vi "Connect.vi"(8 "error in (no error)":errorcluster, 11 "Connection in":refnum<class "Connection.lvclass">) -> (0 "error out":errorcluster, 3 "Connection out":refnum<class "Connection.lvclass">)   [LabVIEW 2013, in "MQTT_Connection.lvlib" / "Connection.lvclass"]
uses:
  Connection.lvclass
  connection notifier.ctl
  Connection.lvclass/Connection.ctl
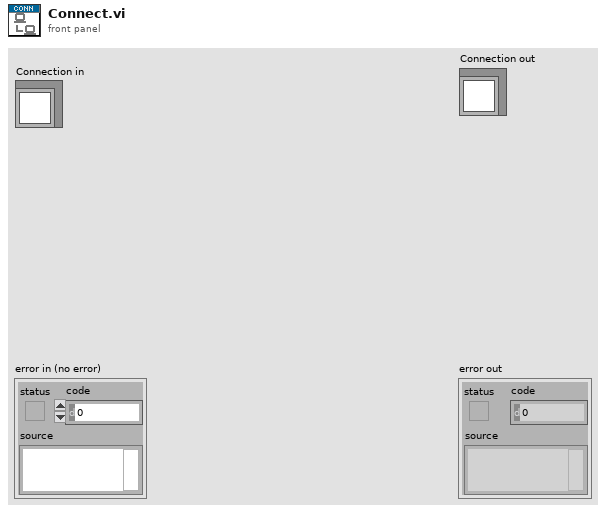
[diagram p1: front panel]
types:
  T1 = typedef "MQTT_Connection.lvlib/Connection.lvclass/connection notifier.ctl" = cluster{"Connection":refnum<class>, "error":errorcluster}
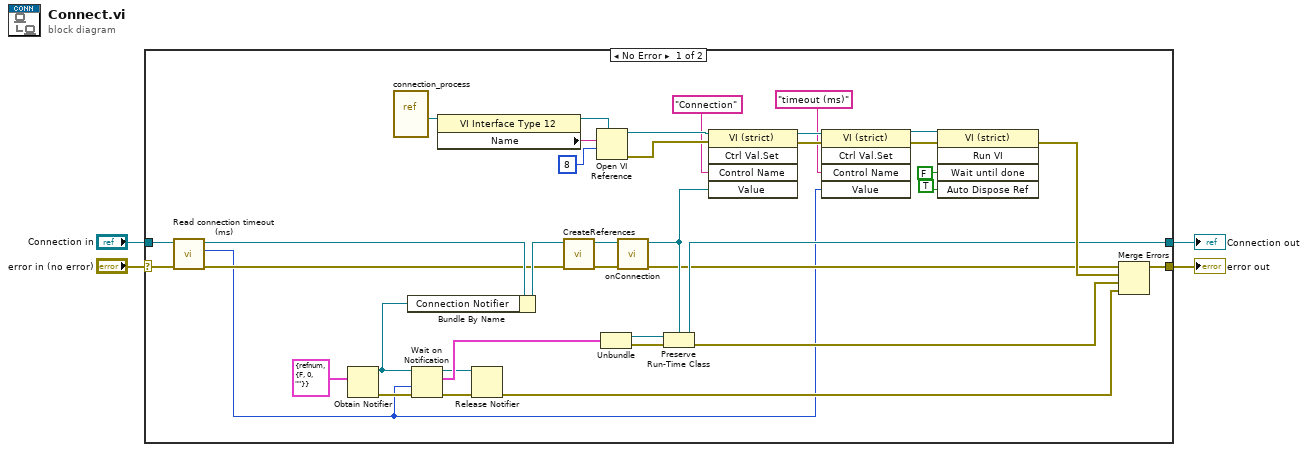
[diagram p0: block diagram]
diagram:
  n1 = case shown="No Error" "error in (no error)" {
    selector: "error in (no error)" -> [w7 w43]
    tunnel: [w39 w43] -> w3
    tunnel: [w14 w42] -> w2
    tunnel: "Connection in" -> [w9 w42]
    frame No Error {
      n2 = call "Read connection timeout (ms).vi"("error in (no error)"=w7, "Connection in"=w9) -> ("error out"=w6:errorcluster, "connection timeout (ms)"=w5:i32, "Connection out"=w8:refnum<class "Connection.lvclass">)  [unwired: 7 in]
      n3 = Obtain Notifier(notification data type=T1 {"Connection"=refnum, "error"={"status"=FALSE, "code"=0, "source"=""}} ("MQTT Server.lvlib:TCPConnection.lvclass:connection notifier")) -> (notifier out=w35:refnum<notifier>, error out=w41:errorcluster)  [unwired: 3 in, 1 out]
      n4 = vi-ref "connection_process.vi"() -> (w38:refnum<vi>)
      n5 = Bundle By Name(cluster=w8, "Connection Notifier"=w35) -> (w18:refnum<class "Connection.lvclass">)
      n6 = Wait on Notification(notifier=w35, timeout in ms (-1)=w5, error in (no error)=w41) -> (notifier out=w31:refnum<notifier>, notification=w40:T1, error out=w33:errorcluster)  [unwired: 1 in, 1 out]
      n7 = property class="VI Interface Type 12"(reference=w38) -> (reference out=w27:refnum<vi>, "Name"=w37:string)  [unwired: 1 in, 1 out]
      n8 = Release Notifier(notifier=w31, error in (no error)=w33) -> (error out=w32:errorcluster)  [unwired: 1 in, 2 out]
      n9 = call-dynamic "CreateReferences.vi"("error in (no error)"=w6, "Connection in"=w18) -> ("error out"=w11:errorcluster, "Connection out"=w13:refnum<class "Connection.lvclass">)  [unwired: 8 in]
      n10 = Open VI Reference(type specifier VI Refnum (for type only)=w27, vi path=w37, options=8) -> (vi reference=w30:refnum<vi>, error out=w29:errorcluster)  [unwired: 3 in]
      n11 = Unbundle(w40) -> ("Connection"=w17:refnum<class>, "error"=w16:errorcluster)
      n12 = call-dynamic "onConnection.vi"("error in (no error)"=w11, "Connection in"=w13) -> ("error out"=w10:errorcluster, "Connection out"=w12:refnum<class "Connection.lvclass">)  [unwired: 8 in]
      n13 = Preserve Run-Time Class(object in=w17, error in=w16, 2:w12) -> (object out=w14:refnum<class "Connection.lvclass">, error out=w15:errorcluster)
      n14 = invoke class="VI (strict)" method="Ctrl Val.Set"(reference=w30, error in=w29, "Control Name"="Connection", "Value"=w12) -> (reference out=w26:refnum<vi>, error out=w25:errorcluster)  [unwired: 1 in, 3 out]
      n15 = invoke class="VI (strict)" method="Ctrl Val.Set"(reference=w26, error in=w25, "Control Name"="timeout (ms)", "Value"=w5) -> (reference out=w24:refnum<vi>, error out=w23:errorcluster)  [unwired: 1 in, 3 out]
      n16 = invoke class="VI (strict)" method="Run VI"(reference=w24, error in=w23, "Wait until done"=FALSE ("Wait Until Done"), "Auto Dispose Ref"=TRUE ("Auto Dispose Reference")) -> (error out=w28:errorcluster)  [unwired: 1 in, 4 out]
      n17 = Merge Errors(w10, w28, w15, w32) -> (w39:errorcluster)
    }
    frame Error {
    }
  }
  "error out" <- w3
  "Connection out" <- w2
